vi "DefendGoalTactic.vi"(7 "First call?":bool=TRUE, 8 "error in (no error)":errorcluster, 9 "Robot":refnum<class "Robot.lvclass">, 10 "Game":refnum<class "Game.lvclass">, 11 "DefendGoalTactic in":refnum<class "DefendGoalTactic.lvclass">) -> (0 "error out":errorcluster, 2 "Robot out":refnum<class "Robot.lvclass">, 3 "DefendGoalTactic out":refnum<class "DefendGoalTactic.lvclass">)   [LabVIEW 2024, in "DefendGoalTactic.lvclass"]
uses:
  DefendGoalTactic.lvclass
  Robot_class/Robot.lvclass
  C:/Users/moise/Documents/GitHub/SSL_AI/Object_class/Object.lvclass
  Game_class/Game.lvclass
  C:/Users/moise/Documents/GitHub/SSL_AI/Tactic_class/Tactic.lvclass
  Robot_class/tactics.ctl
  DefendGoalTacticStates.ctl
  Tactic_class/Tactic.lvclass/Tactic.ctl
  Robot_class/robotKickToStates.ctl
  Robot_class/Robot.lvclass/Robot.ctl
  Game_class/Game.lvclass/Game.ctl
  Parameters_class/Parameters.lvclass/Parameters.ctl
  Team_class/Team.lvclass/Team.ctl
  Field_class/Field.lvclass/Field.ctl
  Object_class/Object.lvclass/Object.ctl
  Skillbook_class/Skillbook.lvclass/Skillbook.ctl
  DefendGoalTactic.lvclass/DefendGoalTactic.ctl
  Robot_class/Write robotKickState.vi
  Object_class/Read position(x,y).vi
  Game_class/Read OffensiveTeam.vi
  Game_class/Read EnemyRef.vi
  Game_class/Read Parameters.lvclass.vi
  Game_class/Read Utilities.lvclass.vi
  Game_class/Read FieldRef.vi
  Game_class/Read BallRef.vi
  Field_class/Read ourGoalPosition.vi
  Parameters_class/Read AttakingOurselves.vi
  Team_class/Read RobotRef.vi
  Robot_class/Write dest_orientation.vi
  Robot_class/Write dest_x.vi
  Robot_class/Write dest_y.vi
  Object_class/Read x.vi
  Object_class/Read y.vi
  Game_class/Read NewParameters.vi
  Skillbook_class/Read KickToSkill.vi
  Robot_class/Write kick_x.vi
  Robot_class/Write kick_z.vi
  Tactic_class/Read Skillbook.vi
  Write States.vi
  Robot_class/Write tactic.vi
  Robot_class/Write keepDest.vi
  Enemy_class/Enemy.lvclass
  C:/Users/moise/Documents/GitHub/SSL_AI/Team_class/Team.lvclass
  Ally_class/Ally.lvclass
  Ball_class/Ball.lvclass
  Skillbook_class/Skillbook.lvclass
  DefBallTrajSkill_class/DefBallTrajSkill.lvclass
  Parameters_class/Parameters.lvclass
  Utilities_class/Utilities.lvclass
  Field_class/Field.lvclass
  KickToSkill_class/KickToSkill.lvclass
  ShootTactic_class/ShootTactic.lvclass
  <vilib>/Analysis/NI_AALPro.lvlib
  <vilib>/Analysis/coordinate.llb/2D Cartesian Coordinate Rotation (Scalar).vi
  Team_class/Team.lvclass
  DefBallEnemySkill_class/DefBallEnemySkill.lvclass
  DefBallOrientSkill_class/DefBallOrientSkill.lvclass
panel:
  out "Dist":dbl
  out "x .or. y?":bool
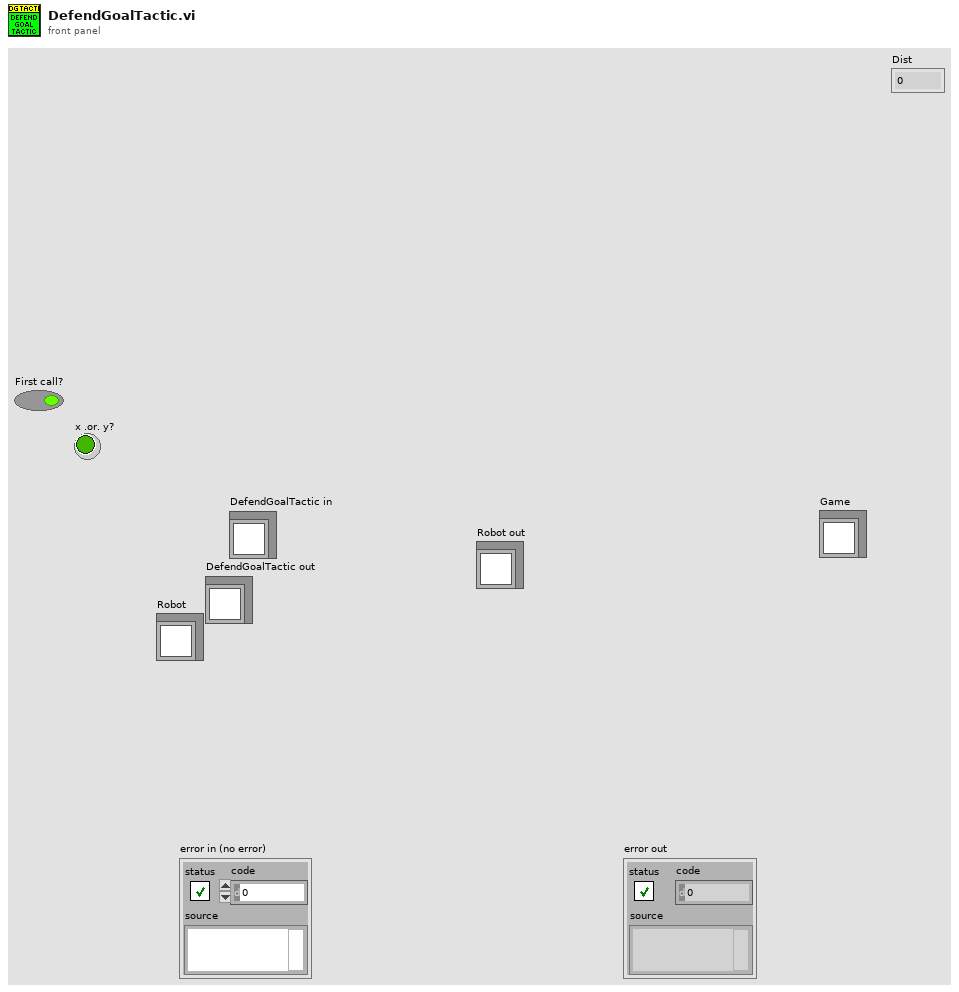
[diagram p1: front panel]
types:
  T1 = typedef "DefendGoalTactic.lvclass/DefendGoalTacticStates.ctl" = enum16{"BlockShot", "BlockPossibleShot", "CoverOneTouchShot", "Kick", "GuardGoal", "Exit"}
  T2 = typedef "tactics.ctl" = enum16{"GoToBallPlacementPosition", "PlaceBall", "GoToBallPlacement", "5Robots", "BallPlacementEnemy", "ReceivePassInFuturePoint", "Roller", "PrepareRollToPassRollerGoTo", "PrepareRollToPassReceiverGoTo", "WaitRoll", "PositionToRoll", "PenaltyAttacker", "PassObserver", "PenaltyDefense", "TableReceiverTactic", "Test", "DefendGoal", "Marker", "FollowAttacker", "DefendArea", "Shoot", "AttackerAimGoal", "AttackerBallOutOfField", "AttackerBlock", "AttackerStop", "Duelist", "Halt", "ZigZag", "GoTo", "Timeout", "KickToBestRobot", "KickToPassReceiver", "PositionToReceivePass", "WaitPass", "GoToTarget"}
  T3 = typedef "robotKickToStates.ctl" = enum16{"shootFromDirect", "avoidCollideBall", "goToBackBall", "none", "walk", "turn", "turnAntiClockWise", "turnClockwise", "oldKickToShoot", "oldKickToGoToBackBall", "shoot"}
  T4 = typedef "NewParameters.ctl" = cluster{"PenaltyDistance":dbl, "DistanceAttackerToBackBall":dbl, "Division":enum16{"Div B", "Div A"}, "DistanceToAvoidyEnemyRobot":dbl, "BallPlacementDistance":dbl, "DisatanceBehindBallToStealBall":dbl, "MaxDistanceToPositionKickoff":dbl, "BlockEnemyTarget":bool, "MaxStopVAng":dbl, "DistanceMarkerToEnemy":dbl, "IgnoreDribblerContact":bool, "DistanceToBeginEnemyPosession":dbl, "GoToBallWhenEnemyNotMoving":bool, "EnemyDistanceToReduceVelocity":dbl, "TurnOnEnemyDistanceToReduceVelocity":bool, "EnemyDistanceToShootOutBall":dbl, "DefenseKickBall":bool, "MoreKickToGoal? (0-0.3)":dbl, "ChipKickInEnemyField":bool, "ShootOutRobotId":dbl, "FieldLenghtDenominatorInShootOut":dbl, "AdjustPositionInBallPlacement":bool, "PowerGodPass":dbl, "VelocityAbortEnemyPos":dbl, "MaxDistToBeginPass":dbl, "MinDistToBeginPass":dbl, "VelocityInDirects":dbl, "BadDribblerIDs":i32[], "NewKickToDistanceAroundBall":dbl, "PowerAvoidColisionMarker":dbl, "DistanceToAvoidColisionMarker":dbl, "AvoidBallKick":dbl, "DistanceTryKick":dbl, "SuicideKickDIstance":dbl, "AdjustFirstKickDistance":dbl, "AvoidAimLessKick":dbl, "DistanceToAvoidyEnemyShootRobot ":dbl, "NumberOfMarkers":dbl, "PotField":bool, "PIDLateral":bool, "MinDistanceFirstKickX":dbl, "MinDistanceFirstKickY":dbl, "FractionOfDistToTouchGround\nAfterChipKick":dbl, "FractionOfKickxWhen\nComposedWithKickz":dbl, "Style":T5, "MoveInTurnState":bool, "DistFromEnemyToConsider\nMoveInTurnState":dbl, "CascadePID":bool, "TurnAroundParameters":cluster{"Radius":dbl, "Multiplier":dbl, "ChordAngle":dbl}, "SafeDriveVel":dbl, "DistanceToGoToBackBall":dbl, "minDistanceToNotFinish\nEnemyPossession":dbl, "OneTouchShot":cluster{"angleFactor":dbl, "maxAngle":dbl, "Attack":bool, "Defense":bool}, "OpenAngleToGoal":cluster{"minAngle":dbl, "maxAngle":dbl, "minEvaluation":dbl}, "ShotInterception":cluster{"shotSpeed":dbl, "minEnemySpeed":dbl, "maxEnemySpeed":dbl, "minEvaluation":dbl}, "AllyTeamArray":T6[], "maxDefendersNumber":i32, "Zone":cluster{"GuardPositionArray":dbl[][], "ZoneMidField":dbl[], "CenterForwardWidth":dbl}, "MinEvaluationToShoot":dbl, "PassInterception":cluster{"maxPassSpeed":dbl, "minPassSpeed":dbl, "minEnemySpeed":dbl, "chipPassDistance":dbl, "chipPassEvaluation":dbl, "minEvaluation":dbl, "maxEnemySpeed":dbl}, "PassDistance":cluster{"maxDistance":dbl, "minDistance":dbl}, "receiverSpeed":dbl, "maxBallSpeed":dbl, "slackTime":dbl, "Turning radius":dbl, "Turning v_ang":dbl, "AlignError":cluster{"Distance":dbl, "Orientation":dbl, "V_norm(m/s)":dbl, "V_ang (rad/s)":dbl}, "RobotRadius":dbl, "KickerDistance":dbl, "keeper angle  to cover goalpost":dbl, "a_slide":dbl, "a_roll":dbl, "k_switch":dbl}
  T5 = typedef "Style.ctl" = enum16{"Insanity", "Offensive", "Defensive"}
  T6 = typedef "AllyTeam.ctl" = enum16{"Keeper", "Defender", "Attacker"}
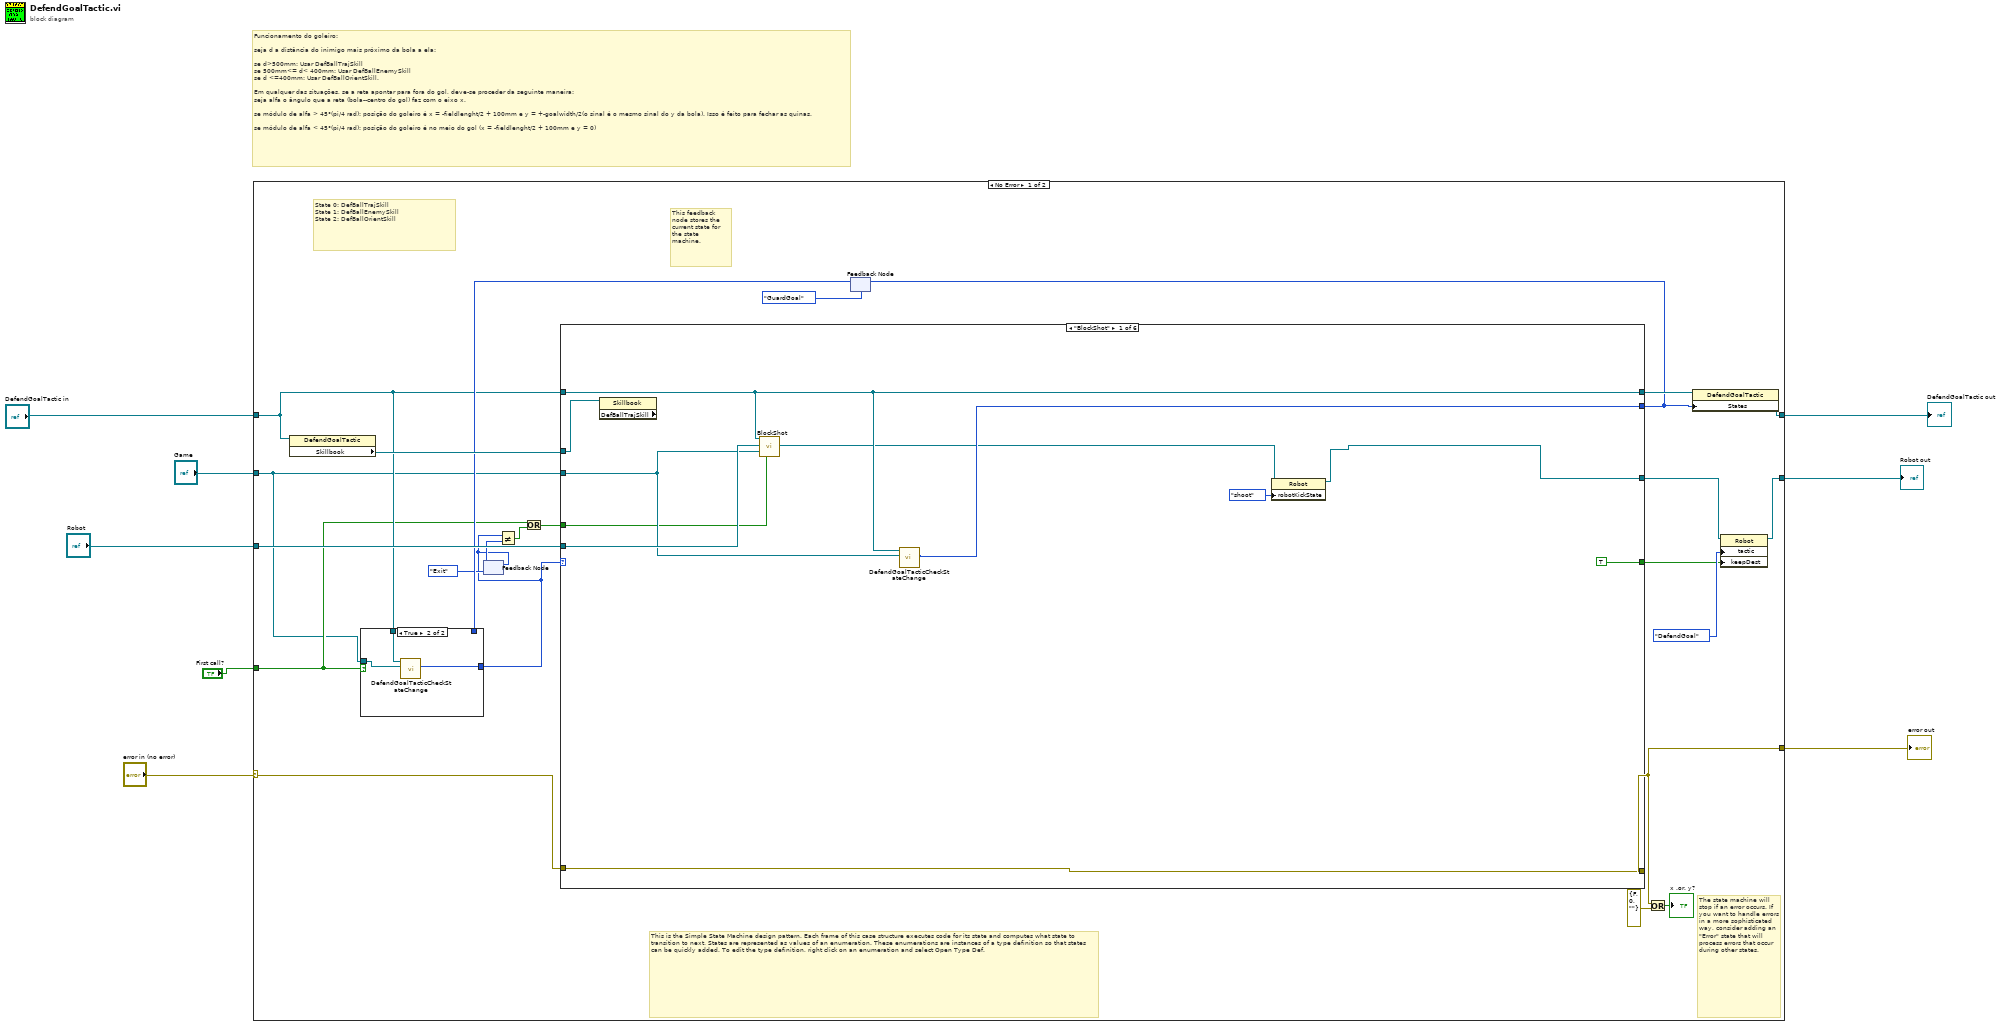
[diagram p0: block diagram]
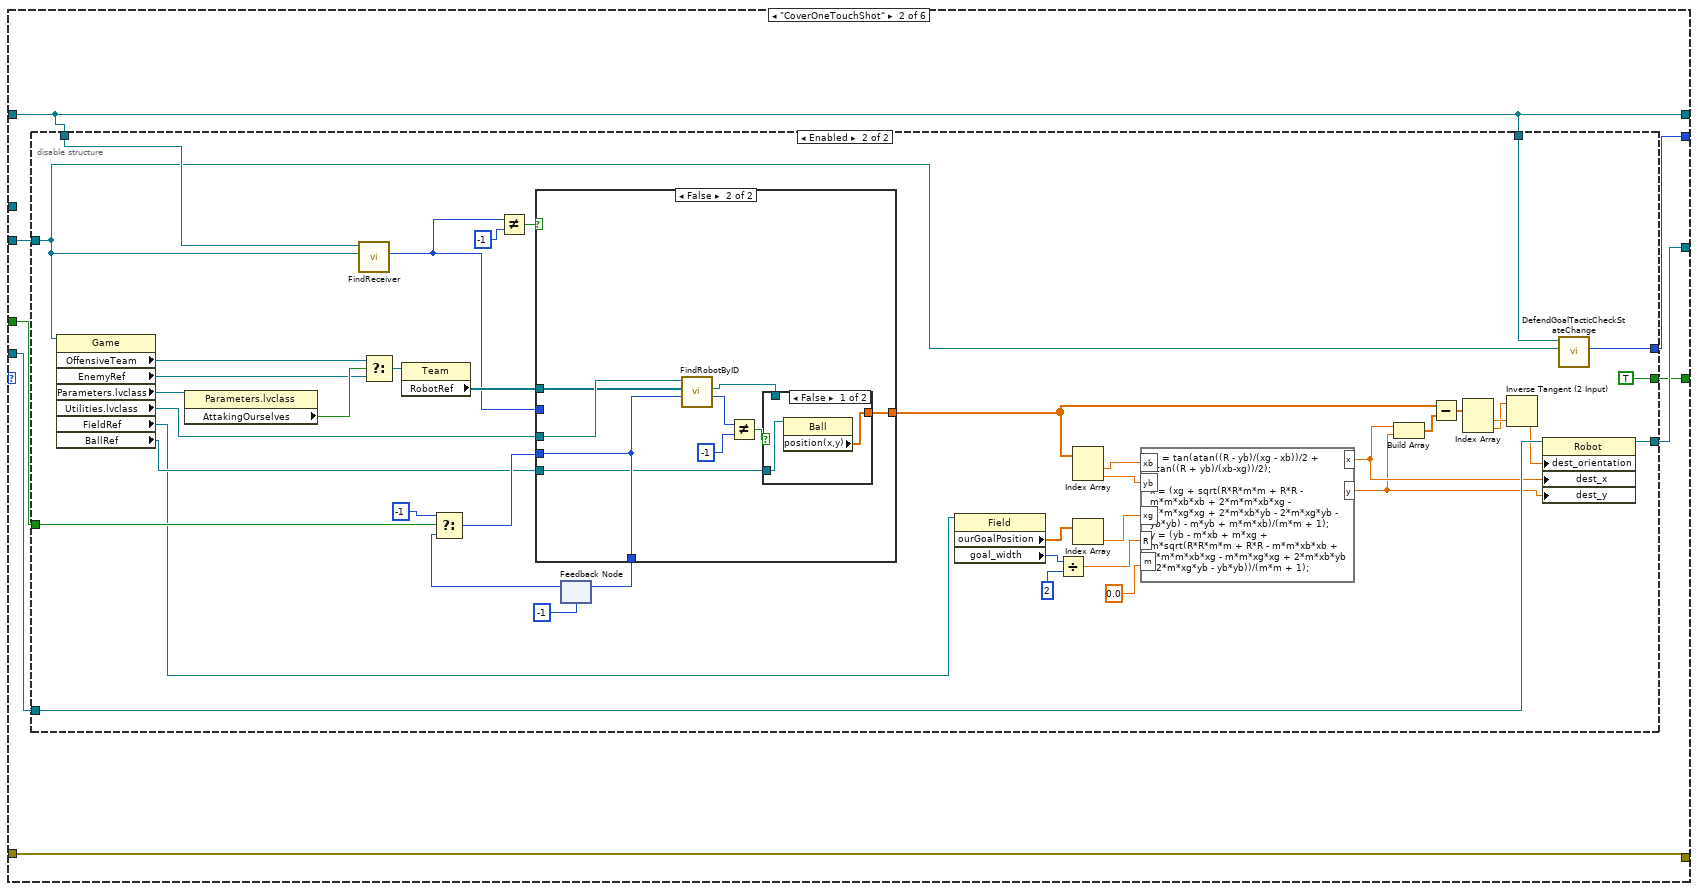
[diagram p3: hidden frame]
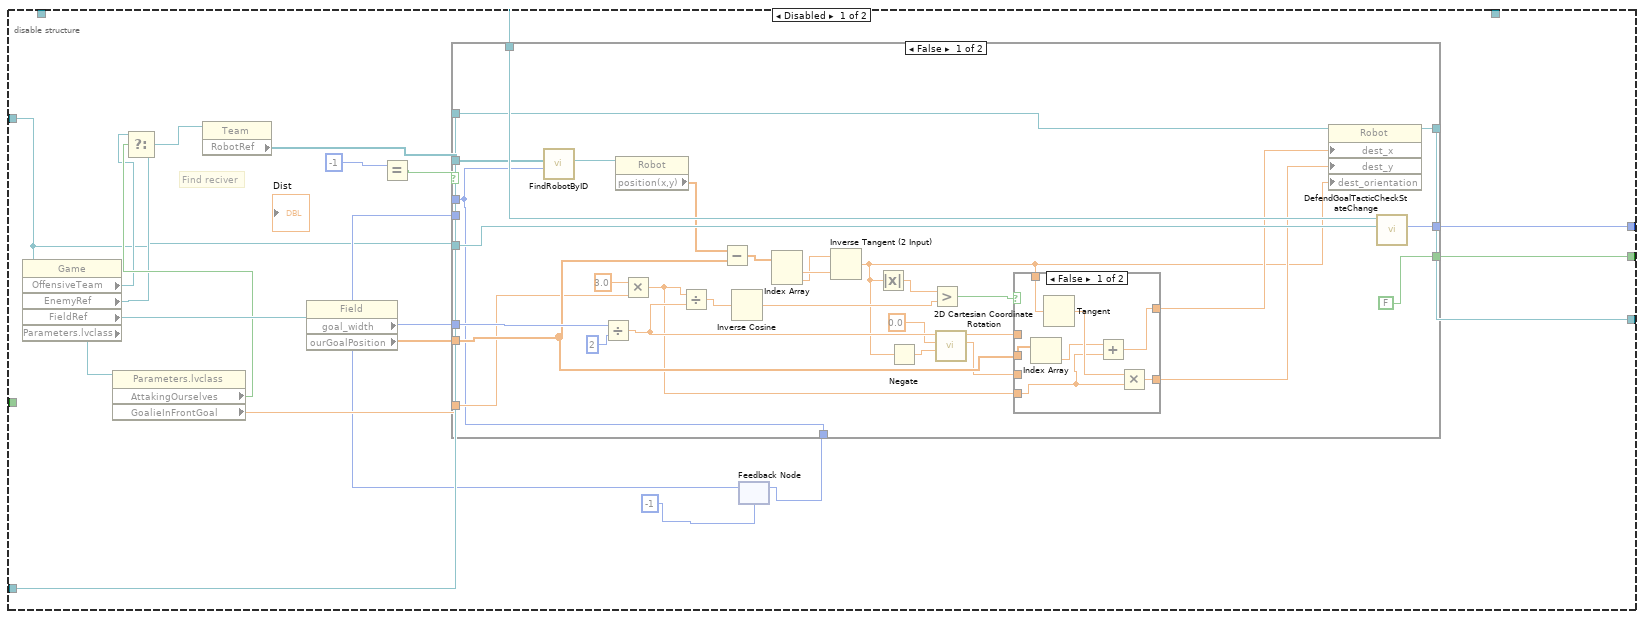
[diagram p4: hidden frame]
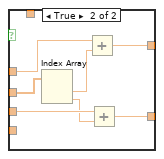
[diagram p5: hidden frame]
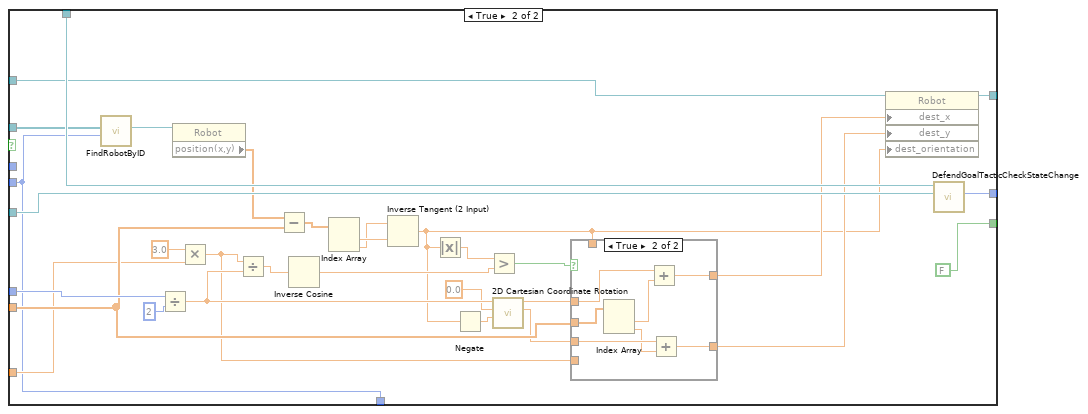
[diagram p6: hidden frame]
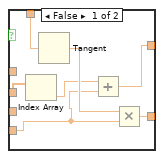
[diagram p7: hidden frame]
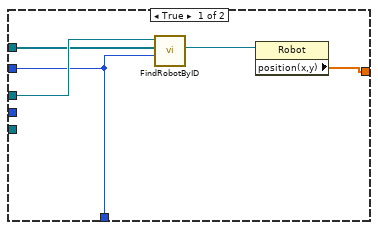
[diagram p8: hidden frame]
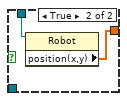
[diagram p9: hidden frame]
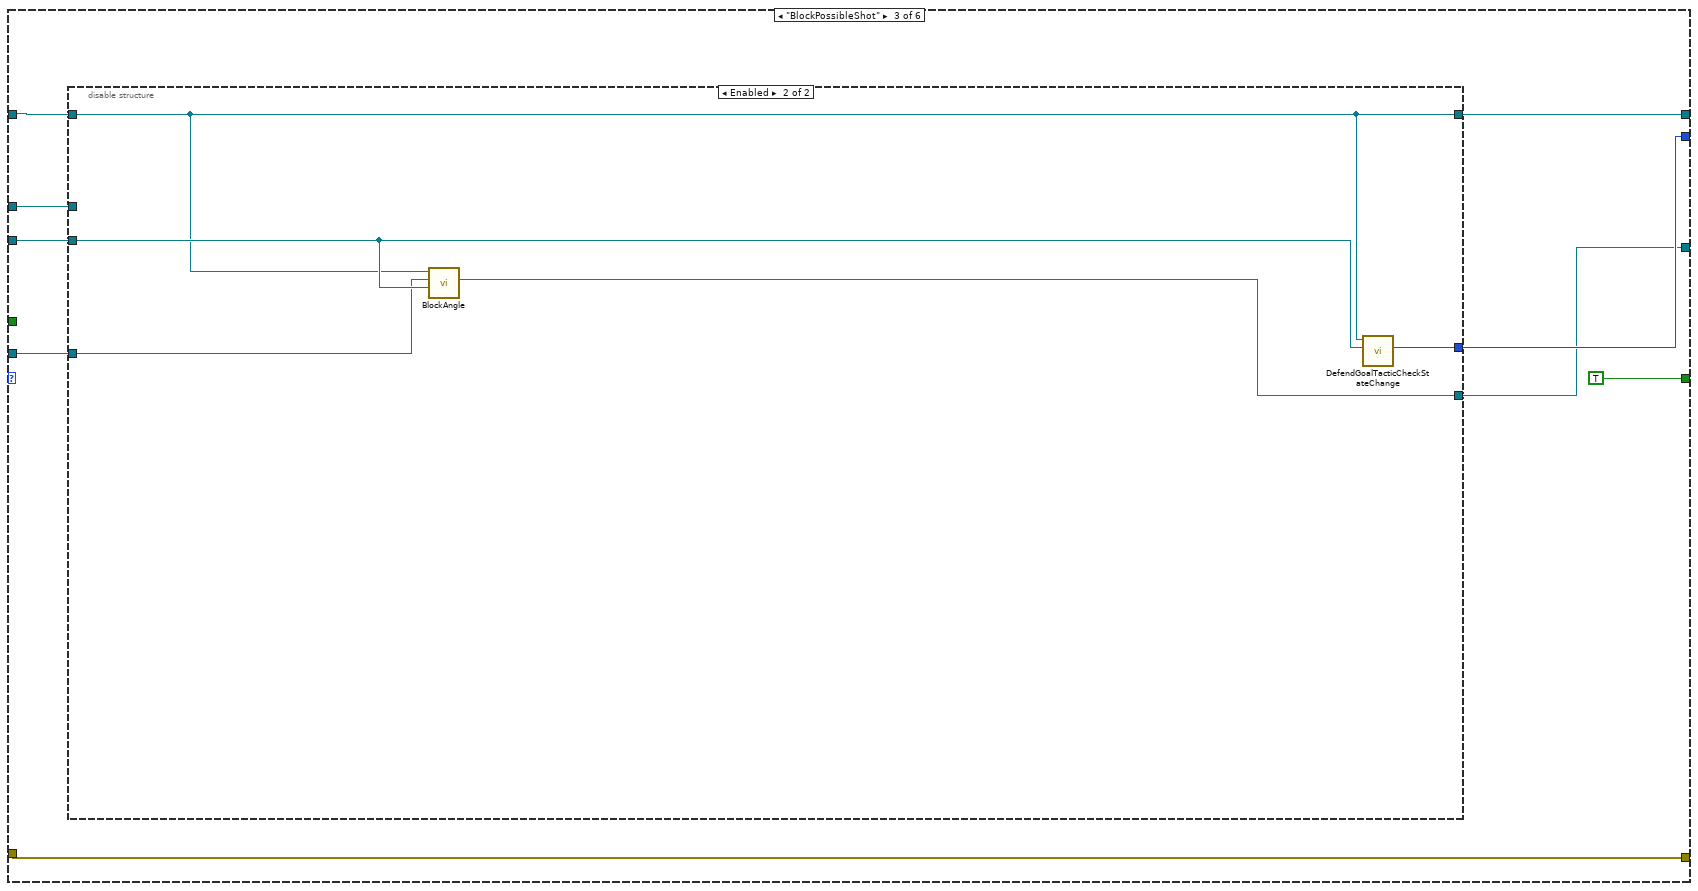
[diagram p10: hidden frame]
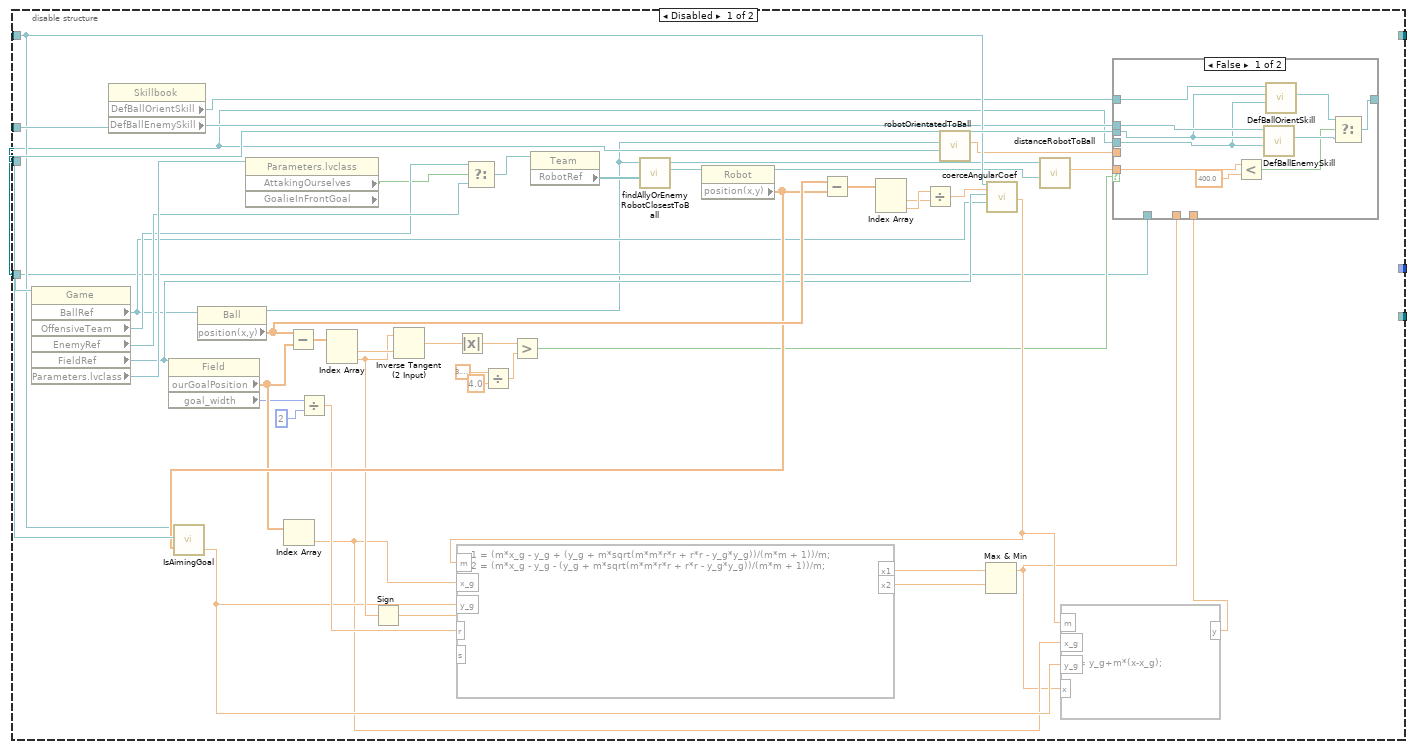
[diagram p11: hidden frame]
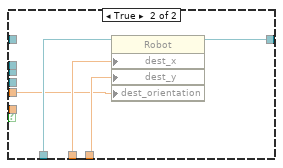
[diagram p12: hidden frame]
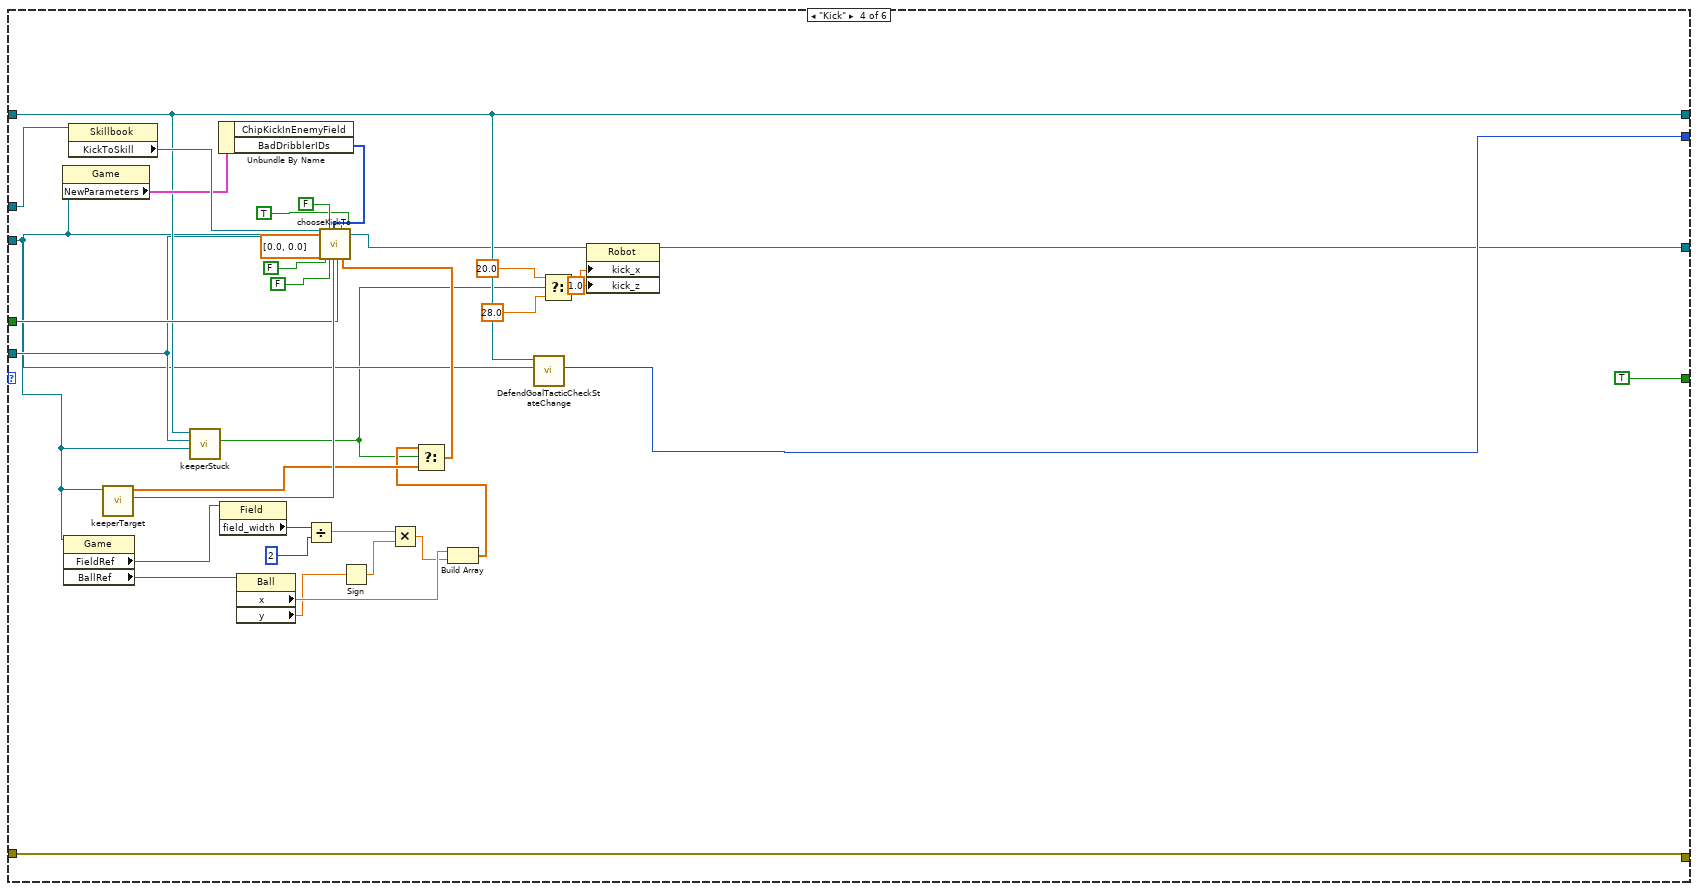
[diagram p13: hidden frame]
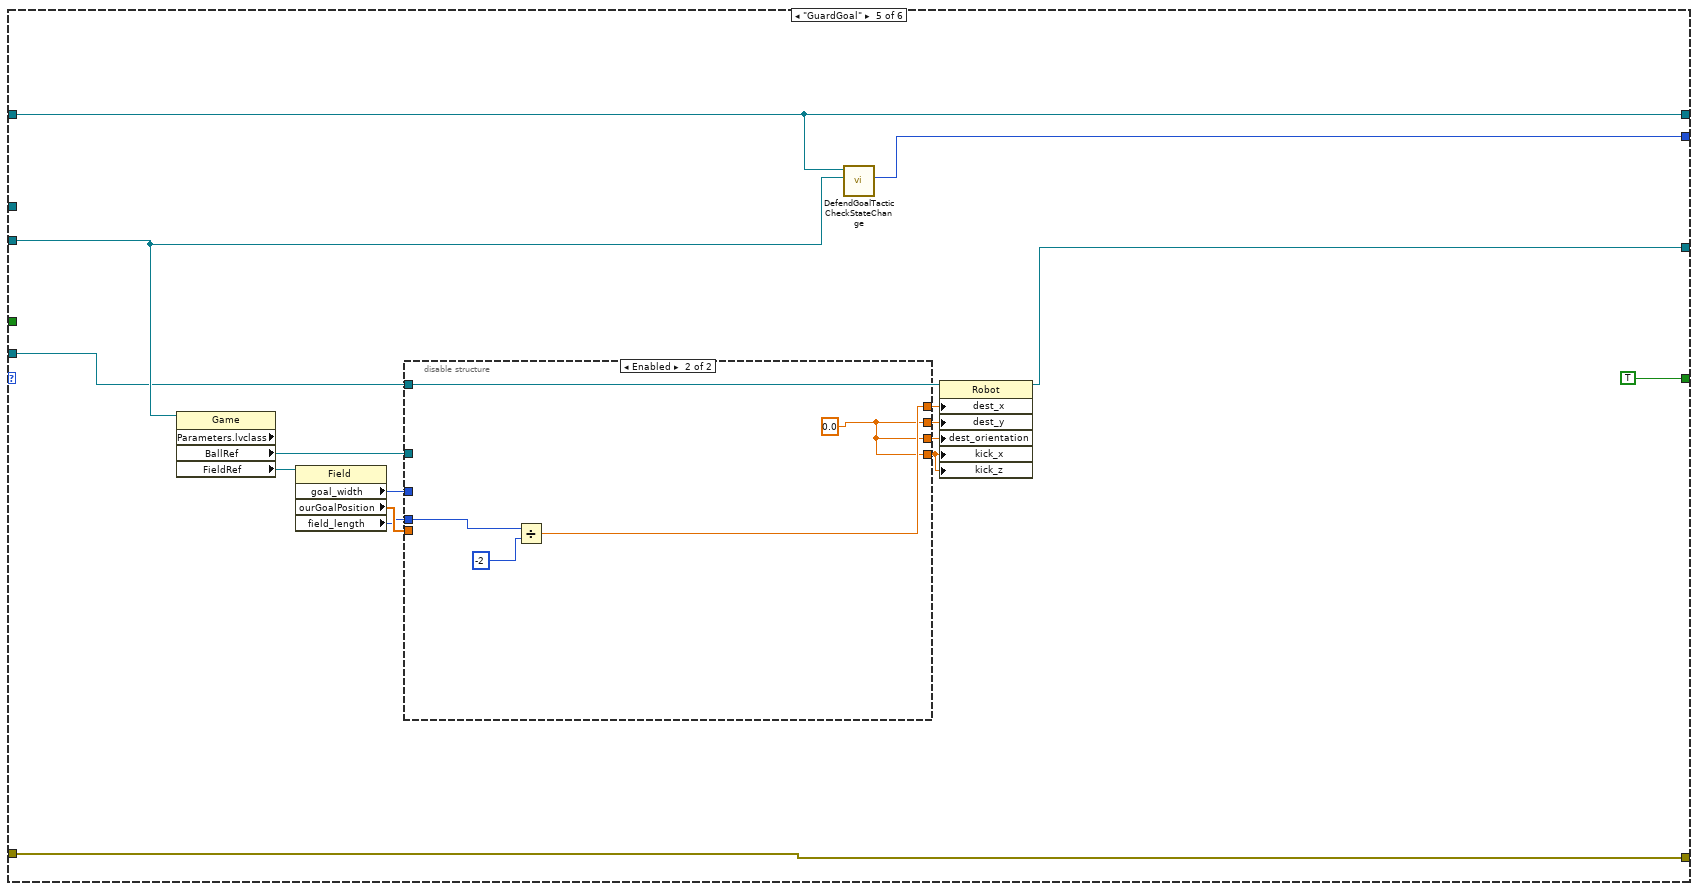
[diagram p14: hidden frame]
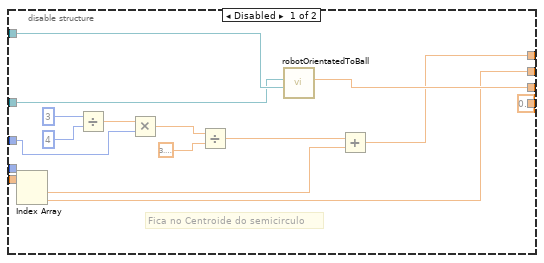
[diagram p15: hidden frame]
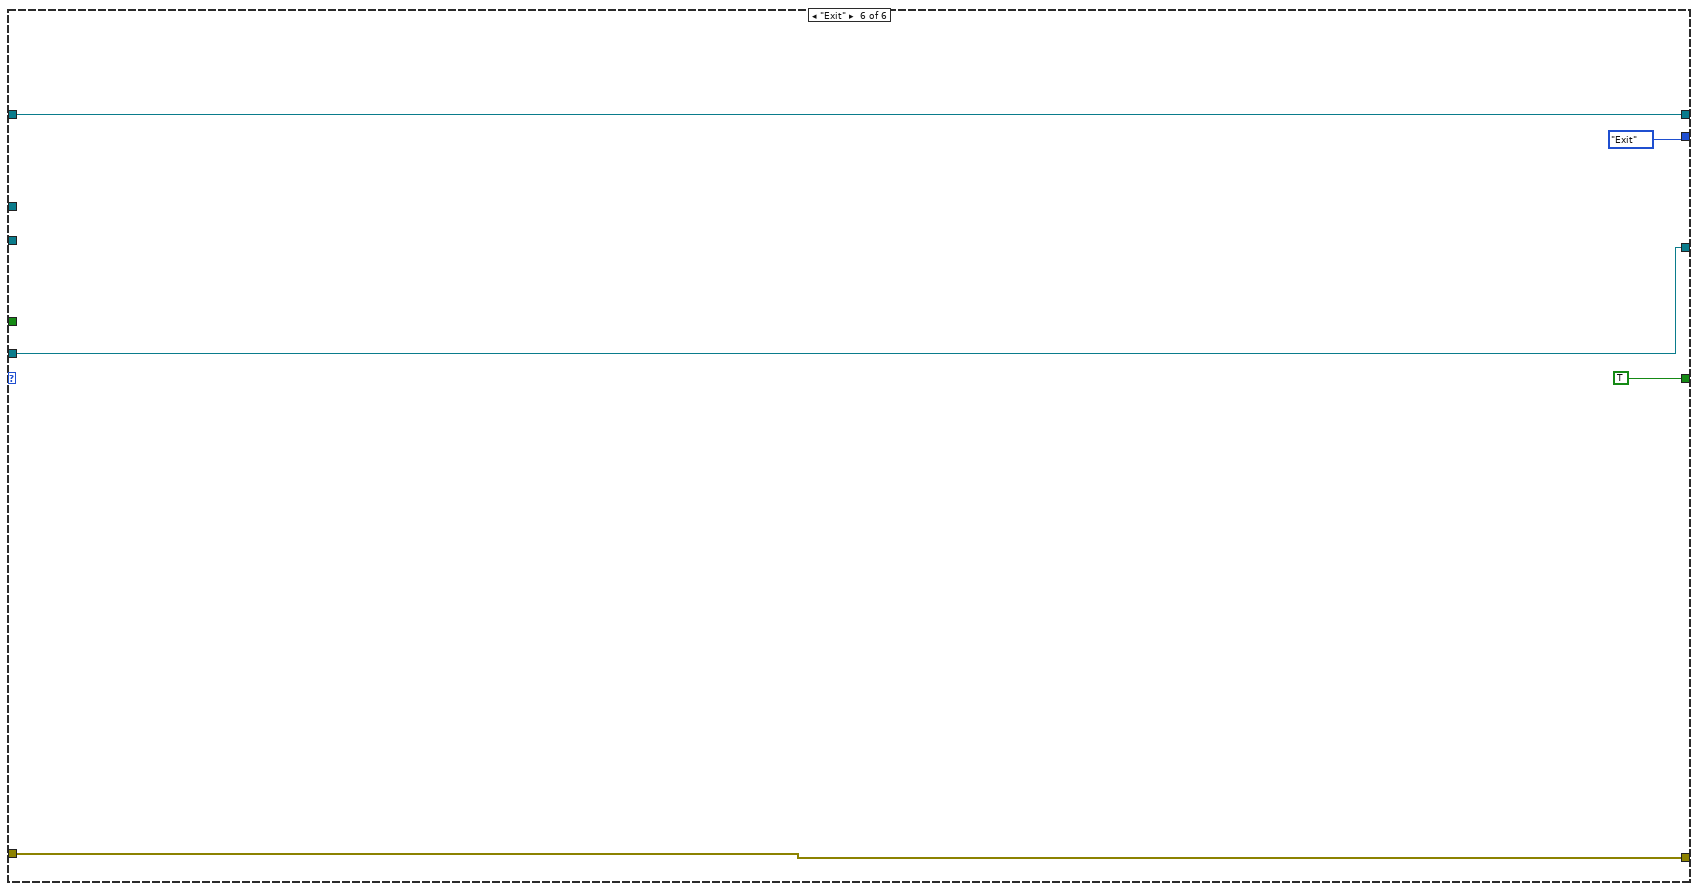
[diagram p16: hidden frame]
diagram:
  # "Funcionamento do goleiro:\n\nseja d a distância do inimigo mais próximo da bola a ela:\n\nse d>500mm: Usar DefBallTrajSkill\nse 500mm<= d< 400mm: Usar DefBallEnemySkill\nse d <=400mm: Usar DefBallOrientSkill.\n\nEm qualquer das situações, se a reta apontar para fora do gol, deve-se proceder da seguinte maneira:\nseja alfa o ângulo que a reta (bola--centro do gol) faz com o eixo x.\n\nse módulo de alfa > 45°(pi/4 rad): posição do goleiro é x = -fieldlenght/2 + 100mm e y = +-goalwidth/2(o sinal é o mesmo sinal do y da bola). Isso é feito para fechar as quinas.\n\nse módulo de alfa < 45°(pi/4 rad): posição do goleiro é no meio do gol (x = -fieldlenght/2 + 100mm e y = 0)"
  n1 = case shown="No Error" "error in (no error)" {
    selector: "error in (no error)" -> [w30 w378]
    tunnel: [w29 w378] -> w7
    tunnel: [w25 w377] -> w2
    tunnel: "DefendGoalTactic in" -> [w22 w377]
    tunnel: "Robot" -> [w28 w376]
    tunnel: [w19 w376] -> w5
    tunnel: "Game" -> [w10 _]
    tunnel: "First call?" -> [w16 _]
    frame No Error {
      # "State 0: DefBallTrajSkill\nState 1: DefBallEnemySkill\nState 2: DefBallOrientSkill"
      # "The state machine will stop if an error occurs. If you want to handle errors in a more sophisticated way, consider adding an \"Error\" state that will process errors that occur during other states."
      # "This feedback node stores the current state for the state machine."
      # "This is the Simple State Machine design pattern. Each frame of this case structure executes code for its state and computes what state to transition to next. States are represented as values of an enumeration. These enumerations are instances of a type definition so that states can be quickly added. To edit the type definition, right click on an enumeration and select Open Type Def."
      n2 = property class="DefendGoalTactic"(reference=w22) -> ("Skillbook"=w27:refnum<class "Skillbook.lvclass">)  [unwired: 1 in, 2 out]
      n3 = feedback #1(DefendGoalTacticStates."Exit" ("States")) -> (w14:T1)
      n4 = feedback #2(DefendGoalTacticStates."GuardGoal" ("States")) -> (w24:T1)
      n5 = case shown="True" w16 {
        tunnel: [w32 w35] -> w9
        tunnel: w24 -> [w32 _]
        tunnel: w10 -> [_ w34]
        tunnel: w22 -> [_ w33]
        frame False {
        }
        frame True {
          n6 = call "DefendGoalTacticCheckStateChange.vi"("Game"=w34, "DefendGoalTactic in"=w33) -> ("States"=w35:T1)  [unwired: 7 in, 2 out]
        }
      }
      n7 = feedback-in #1(w9) -> ()
      n8 = Not Equal?(x=w9, y=w14) -> (x != y?=w15:bool)
      n9 = Or(x=w16, y=w15) -> (x .or. y?=w17:bool)
      n10 = case shown="\"BlockShot\"" w9 {
        tunnel: w30 -> [w46 w54 w233 w335 w351 w375]
        tunnel: [w46 w54 w233 w335 w351 w375] -> w29
        tunnel: w27 -> [w45 _ w232 w333 _ _]
        tunnel: w28 -> [w41 w51 w230 w320 w346 w371]
        tunnel: [w37 w52 w227 w306 w344 w371] -> w20
        tunnel: [w42 w48 w225 w324 w349 w372] -> w26
        tunnel: w22 -> [w42 w48 w229 w324 w349 w372]
        tunnel: w10 -> [w40 w53 w231 w319 w348 _]
        tunnel: [w44 w49 w228 w308 w350 DefendGoalTacticStates."Exit" ("States")] -> w18
        tunnel: w17 -> [w39 w47 _ w329 _ _]
        tunnel: [TRUE ("keepDest") w50 TRUE TRUE ("keepDest") TRUE ("keepDest") TRUE ("keepDest")] -> w11
        frame "BlockShot" {
          n11 = property class="Skillbook" props=["DefBallTrajSkill"](reference=w45) -> ()  [unwired: 1 in, 3 out]
          n12 = call "BlockShot.vi"("object in"=w42, "Robot"=w41, "Game"=w40, "first call?"=w39) -> ("Robot out"=w38:refnum<class "Robot.lvclass">)  [unwired: 13 in, 2 out]
          n13 = call "DefendGoalTacticCheckStateChange.vi"("Game"=w40, "DefendGoalTactic in"=w42) -> ("States"=w44:T1)  [unwired: 7 in, 2 out]
          n14 = property class="Robot"(reference=w38, "robotKickState"=robotKickToStates."shoot") -> (reference out=w37:refnum<class "Robot.lvclass">)  [unwired: 1 in, 1 out]
        }
        frame "CoverOneTouchShot" {
          n15 = disable-structure shown="Enabled" {
            disable-tunnel: w48 -> [w75 w202]
            disable-tunnel: w53 -> [w55 w191]
            disable-tunnel: [w73 w186] -> w52
            disable-tunnel: w51 -> [w72 w173]
            disable-tunnel: [w67 w195] -> w49
            disable-tunnel: [w63 TRUE ("keepDest")] -> w50
            disable-tunnel: w48 -> [_ w194]
            disable-tunnel: w47 -> [_ w190]
            frame Disabled {
              # "Find reciver"
              n16 = property class="Game"(reference=w55) -> ("OffensiveTeam"=w56:refnum<class "Ally.lvclass">, "EnemyRef"=w57:refnum<class "Enemy.lvclass">, "FieldRef"=w71:refnum<class "Field.lvclass">, "Parameters.lvclass"=w65:refnum<class "Parameters.lvclass">)  [unwired: 1 in, 2 out]
              n17 = property class="Parameters.lvclass"(reference=w65) -> ("AttakingOurselves"=w59:bool, "GoalieInFrontGoal"=w64:dbl)  [unwired: 1 in, 2 out]
              n18 = Select(t=w56, s=w59, f=w57) -> (s? t:f=w58:refnum<class "Team.lvclass">)
              n19 = property class="Team"(reference=w58) -> ("RobotRef"=w74:refnum<class "Robot.lvclass">[])  [unwired: 1 in, 2 out]
              n20 = property class="Field"(reference=w71) -> ("goal_width"=w66:i32, "ourGoalPosition"=w70:dbl[])  [unwired: 1 in, 2 out]
              n21 = Equal?(x=-1) -> (x = y?=w68:bool)  [unwired: 1 in]
              n22 = feedback #3(-1 ("x")) -> (w61:i32)
              n23 = case shown="False" w68 {
                tunnel: w75 -> [w106 w151]
                tunnel: w55 -> [w105 w150]
                tunnel: w74 -> [w104 w149]
                tunnel: [w103 w148] -> w73
                tunnel: w72 -> [w102 w147]
                tunnel: w70 -> [w86 w131]
                tunnel: [w100 w145] -> w67
                tunnel: w66 -> [w95 w140]
                tunnel: w64 -> [w84 w129]
                tunnel: _ -> [w78 _]
                tunnel: [FALSE ("keepDest") FALSE ("keepDest")] -> w63
                tunnel: w61 -> [_ w123]
                tunnel: [w78 w123] -> w60
                frame False {
                  n24 = call "FindRobotByID.vi"("id"=w78, "RobotRef"=w104) -> ("Robot"=w101:refnum<class "Robot.lvclass">)  [unwired: 6 in, 3 out]
                  n25 = Divide(x=w95, y=2) -> (x/y=w88:dbl)
                  n26 = property class="Robot"(reference=w101) -> ("position(x,y)"=w99:dbl[])  [unwired: 1 in, 2 out]
                  n27 = Multiply(x=3.0, y=w84) -> (x*y=w80:dbl)
                  n28 = Divide(x=w80, y=w88) -> (x/y=w92:dbl)
                  n29 = Subtract(x=w99, y=w86) -> (x-y=w98:dbl[])
                  n30 = Inverse Cosine(1:w92) -> (0:w91:dbl)
                  n31 = Index Array(array=w98) -> (element #1=w97:dbl, element #2=w96:dbl)  [unwired: 2 in]
                  n32 = Inverse Tangent (2 Input)(1:w97, 2:w96) -> (0:w77:dbl)
                  n33 = Absolute Value(x=w77) -> (abs(x)=w90:dbl)
                  n34 = Negate(x=w77) -> (-x=w76:dbl)
                  n35 = Greater?(x=w90, y=w91) -> (0:w89:bool)
                  n36 = call-poly <vilib>:"2D Cartesian Coordinate Rotation.vi"("theta"=w76, "y"=0.0 ("element"), "x"=w88) -> ("y out"=w83:dbl, "x out"=w85:dbl)  [unwired: 6 in, 1 out]
                  n37 = case shown="False" w89 {
                    tunnel: w86 -> [w110 w118]
                    tunnel: w85 -> [_ w120]
                    tunnel: w83 -> [_ w119]
                    tunnel: [w107 w115] -> w82
                    tunnel: [w111 w114] -> w81
                    tunnel: w80 -> [w108 _]
                    tunnel: w77 -> [w113 _]
                    frame False {
                      n38 = Index Array(array=w110) -> (element=w109:dbl)  [unwired: 1 in]
                      n39 = Tangent(1:w113) -> (0:w112:dbl)
                      n40 = Add(x=w109, y=w108) -> (x+y=w107:dbl)
                      n41 = Multiply(x=w112, y=w108) -> (x*y=w111:dbl)
                    }
                    frame True {
                      n42 = Index Array(array=w118) -> (element #1=w117:dbl, element #2=w116:dbl)  [unwired: 2 in]
                      n43 = Add(x=w120, y=w117) -> (x+y=w115:dbl)
                      n44 = Add(x=w119, y=w116) -> (x+y=w114:dbl)
                    }
                  }
                  n45 = property class="Robot"(reference=w102, "dest_x"=w82, "dest_y"=w81, "dest_orientation"=w77) -> (reference out=w103:refnum<class "Robot.lvclass">)  [unwired: 1 in, 1 out]
                  n46 = call "DefendGoalTacticCheckStateChange.vi"("Game"=w105, "DefendGoalTactic in"=w106) -> ("States"=w100:T1)  [unwired: 7 in, 2 out]
                }
                frame True {
                  n47 = call "FindRobotByID.vi"("id"=w123, "RobotRef"=w149) -> ("Robot"=w146:refnum<class "Robot.lvclass">)  [unwired: 6 in, 3 out]
                  n48 = Divide(x=w140, y=2) -> (x/y=w133:dbl)
                  n49 = property class="Robot"(reference=w146) -> ("position(x,y)"=w144:dbl[])  [unwired: 1 in, 2 out]
                  n50 = Multiply(x=3.0, y=w129) -> (x*y=w125:dbl)
                  n51 = Divide(x=w125, y=w133) -> (x/y=w137:dbl)
                  n52 = Subtract(x=w144, y=w131) -> (x-y=w143:dbl[])
                  n53 = Inverse Cosine(1:w137) -> (0:w136:dbl)
                  n54 = Index Array(array=w143) -> (element #1=w142:dbl, element #2=w141:dbl)  [unwired: 2 in]
                  n55 = Inverse Tangent (2 Input)(1:w142, 2:w141) -> (0:w122:dbl)
                  n56 = Absolute Value(x=w122) -> (abs(x)=w135:dbl)
                  n57 = Negate(x=w122) -> (-x=w121:dbl)
                  n58 = Greater?(x=w135, y=w136) -> (0:w134:bool)
                  n59 = call-poly <vilib>:"2D Cartesian Coordinate Rotation.vi"("theta"=w121, "y"=0.0 ("element"), "x"=w133) -> ("y out"=w128:dbl, "x out"=w130:dbl)  [unwired: 6 in, 1 out]
                  n60 = case shown="True" w134 {
                    tunnel: w131 -> [w155 w163]
                    tunnel: w130 -> [_ w165]
                    tunnel: w128 -> [_ w164]
                    tunnel: [w152 w160] -> w127
                    tunnel: [w156 w159] -> w126
                    tunnel: w125 -> [w153 _]
                    tunnel: w122 -> [w158 _]
                    frame False {
                      n61 = Index Array(array=w155) -> (element=w154:dbl)  [unwired: 1 in]
                      n62 = Tangent(1:w158) -> (0:w157:dbl)
                      n63 = Add(x=w154, y=w153) -> (x+y=w152:dbl)
                      n64 = Multiply(x=w157, y=w153) -> (x*y=w156:dbl)
                    }
                    frame True {
                      n65 = Index Array(array=w163) -> (element #1=w162:dbl, element #2=w161:dbl)  [unwired: 2 in]
                      n66 = Add(x=w165, y=w162) -> (x+y=w160:dbl)
                      n67 = Add(x=w164, y=w161) -> (x+y=w159:dbl)
                    }
                  }
                  n68 = property class="Robot"(reference=w147, "dest_x"=w127, "dest_y"=w126, "dest_orientation"=w122) -> (reference out=w148:refnum<class "Robot.lvclass">)  [unwired: 1 in, 1 out]
                  n69 = call "DefendGoalTacticCheckStateChange.vi"("Game"=w150, "DefendGoalTactic in"=w151) -> ("States"=w145:T1)  [unwired: 7 in, 2 out]
                }
              }
              n70 = feedback-in #3(w60) -> ()
            }
            frame Enabled {
              n71 = property class="Game"(reference=w191) -> ("OffensiveTeam"=w204:refnum<class "Ally.lvclass">, "EnemyRef"=w203:refnum<class "Enemy.lvclass">, "Parameters.lvclass"=w206:refnum<class "Parameters.lvclass">, "Utilities.lvclass"=w201:refnum<class "Utilities.lvclass">, "FieldRef"=w171:refnum<class "Field.lvclass">, "BallRef"=w172:refnum<class "Ball.lvclass">)  [unwired: 1 in, 2 out]
              n72 = property class="Parameters.lvclass"(reference=w206) -> ("AttakingOurselves"=w205:bool)  [unwired: 1 in, 2 out]
              n73 = call "FindReceiver.vi"("Game"=w191, "object in"=w202) -> ("Receiver Id"=w197:i32)  [unwired: 6 in, 3 out]
              n74 = Select(t=w204, s=w205, f=w203) -> (s? t:f=w200:refnum<class "Team.lvclass">)
              n75 = property class="Team"(reference=w200) -> ("RobotRef"=w199:refnum<class "Robot.lvclass">[])  [unwired: 1 in, 2 out]
              n76 = Not Equal?(x=w197, y=-1) -> (x != y?=w198:bool)
              n77 = feedback #4(-1 ("Receiver Id")) -> (w188:i32)
              n78 = Select(t=-1 ("Receiver Id"), s=w190, f=w188) -> (s? t:f=w187:i32)
              n79 = case shown="False" w198 {
                tunnel: w197 -> [w209 _]
                tunnel: w201 -> [w211 w220]
                tunnel: w199 -> [w210 w219]
                tunnel: [w209 w218] -> w193
                tunnel: w187 -> [_ w218]
                tunnel: [w207 w213] -> w167
                tunnel: w172 -> [_ w212]
                frame True {
                  n80 = call "FindRobotByID.vi"("id"=w209, "RobotRef"=w210, "Utilities in"=w211) -> ("Robot"=w208:refnum<class "Robot.lvclass">)  [unwired: 5 in, 3 out]
                  n81 = property class="Robot"(reference=w208) -> ("position(x,y)"=w207:dbl[])  [unwired: 1 in, 2 out]
                }
                frame False {
                  n82 = call "FindRobotByID.vi"("id"=w218, "RobotRef"=w219, "Utilities in"=w220) -> ("index"=w216:i32, "Robot"=w214:refnum<class "Robot.lvclass">)  [unwired: 5 in, 2 out]
                  n83 = Not Equal?(x=w216, y=-1) -> (x != y?=w217:bool)
                  n84 = case shown="False" w217 {
                    tunnel: w214 -> [_ w224]
                    tunnel: [w221 w223] -> w213
                    tunnel: w212 -> [w222 _]
                    frame False {
                      n85 = property class="Ball"(reference=w222) -> ("position(x,y)"=w221:dbl[])  [unwired: 1 in, 2 out]
                    }
                    frame True {
                      n86 = property class="Robot"(reference=w224) -> ("position(x,y)"=w223:dbl[])  [unwired: 1 in, 2 out]
                    }
                  }
                }
              }
              n87 = feedback-in #4(w193) -> ()
              n88 = property class="Field"(reference=w171) -> ("ourGoalPosition"=w183:dbl[], "goal_width"=w181:i32)  [unwired: 1 in, 2 out]
              n89 = Divide(x=w181, y=2) -> (x/y=w179:dbl)
              n90 = Index Array(array=w167) -> (element #1=w185:dbl, element #2=w184:dbl)  [unwired: 2 in]
              n91 = Index Array(array=w183) -> (element=w182:dbl)  [unwired: 1 in]
              n92 = formula code="m = tan(atan((R - yb)/(xg - xb))/2 + atan((R + yb)/(xb-xg))/2);\n\nx = (xg + sqrt(R*R*m*m + R*R - m*m*xb*xb + 2*m*m*xb*xg - m*m*xg*xg + 2*m*xb*yb - 2*m*xg*yb - yb*yb) - m*yb + m*m*xb)/(m*m + 1);\ny = (yb - m*xb + m*xg + m*sqrt(R*R*m*m + R*R - m*m*xb*xb + 2*m*m*xb*xg - m*m*xg*xg + 2*m*xb*yb - 2*m*xg*yb - yb*yb))/(m*m + 1);"("xb"=w185, "yb"=w184, "xg"=w182, "R"=w179, "m"=0.0 ("input variable")) -> ("x"=w169:dbl, "y"=w168:dbl)
              n93 = Build Array(w169, w168) -> (w178:dbl[])
              n94 = Subtract(x=w167, y=w178) -> (x-y=w177:dbl[])
              n95 = Index Array(array=w177) -> (element #1=w176:dbl, element #2=w175:dbl)  [unwired: 2 in]
              n96 = Inverse Tangent (2 Input)(1:w176, 2:w175) -> (0:w170:dbl)
              n97 = property class="Robot"(reference=w173, "dest_orientation"=w170, "dest_x"=w169, "dest_y"=w168) -> (reference out=w186:refnum<class "Robot.lvclass">)  [unwired: 1 in, 1 out]
              n98 = call "DefendGoalTacticCheckStateChange.vi"("Game"=w191, "DefendGoalTactic in"=w194) -> ("States"=w195:T1)  [unwired: 7 in, 2 out]
            }
          }
        }
        frame "BlockPossibleShot" {
          n99 = disable-structure shown="Enabled" {
            disable-tunnel: w232 -> [w275 _]
            disable-tunnel: w231 -> [w261 w298]
            disable-tunnel: w229 -> [w251 w296]
            disable-tunnel: w230 -> [w239 w297]
            disable-tunnel: [_ w299] -> w228
            disable-tunnel: [_ w295] -> w227
            disable-tunnel: [_ w296] -> w225
            frame Disabled {
              n100 = property class="Game"(reference=w261) -> ("BallRef"=w249:refnum<class "Ball.lvclass">, "OffensiveTeam"=w276:refnum<class "Ally.lvclass">, "EnemyRef"=w277:refnum<class "Enemy.lvclass">, "FieldRef"=w250:refnum<class "Field.lvclass">, "Parameters.lvclass"=w279:refnum<class "Parameters.lvclass">)  [unwired: 1 in, 2 out]
              n101 = property class="Skillbook"(reference=w275) -> ("DefBallOrientSkill"=w238:refnum<class "DefBallOrientSkill.lvclass">, "DefBallEnemySkill"=w240:refnum<class "DefBallEnemySkill.lvclass">)  [unwired: 1 in, 2 out]
              n102 = property class="Field"(reference=w250) -> ("ourGoalPosition"=w259:dbl[], "goal_width"=w258:i32)  [unwired: 1 in, 2 out]
              n103 = property class="Ball"(reference=w249) -> (reference out=w236:refnum<class "Ball.lvclass">, "position(x,y)"=w265:dbl[])  [unwired: 1 in, 1 out]
              n104 = property class="Parameters.lvclass" props=["AttakingOurselves", "GoalieInFrontGoal"](reference=w279) -> ("AttakingOurselves"=w274:bool)  [unwired: 1 in, 3 out]
              n105 = Index Array(array=w259) -> (element=w245:dbl)  [unwired: 1 in]
              n106 = Subtract(x=w265, y=w259) -> (x-y=w273:dbl[])
              n107 = Divide(x=w258, y=2) -> (x/y=w256:dbl)
              n108 = Index Array(array=w273) -> (element #1=w254:dbl, element #2=w253:dbl)  [unwired: 2 in]
              n109 = Sign(1:w253) -> (0:w255:dbl)
              n110 = Inverse Tangent (2 Input)(1:w254, 2:w253) -> (0:w268:dbl)
              n111 = Absolute Value(x=w268) -> (abs(x)=w272:dbl)
              n112 = Select(t=w276, s=w274, f=w277) -> (s? t:f=w278:refnum<class "Team.lvclass">)
              n113 = Divide(x=3.141592653589793, y=4.0) -> (x/y=w269:dbl)
              n114 = Greater?(x=w272, y=w269) -> (0:w241:bool)
              n115 = property class="Team"(reference=w278) -> ("RobotRef"=w267:refnum<class "Robot.lvclass">[])  [unwired: 1 in, 2 out]
              n116 = call "findAllyOrEnemyRobotClosestToBall.vi"("Ally/Enemy Robots"=w267, "Ball"=w236) -> ("Robot"=w266:refnum<class "Robot.lvclass">)  [unwired: 5 in, 4 out]
              n117 = property class="Robot"(reference=w266) -> (reference out=w237:refnum<class "Robot.lvclass">, "position(x,y)"=w260:dbl[])  [unwired: 1 in, 1 out]
              n118 = call "IsAimingGoal.vi"("object in"=w251, "Game"=w261, "Robot position"=w260) -> ("Y aiming in goal coerced"=w246:dbl)  [unwired: 13 in, 3 out]
              n119 = Subtract(x=w265, y=w260) -> (x-y=w264:dbl[])
              n120 = Index Array(array=w264) -> (element #1=w262:dbl, element #2=w263:dbl)  [unwired: 2 in]
              n121 = Divide(x=w263, y=w262) -> (x/y=w252:dbl)
              n122 = call "robotOrientatedToBall.vi"("Robot"=w239, "BallRef"=w236) -> ("Orientation"=w234:dbl)  [unwired: 7 in, 2 out]
              n123 = call "coerceAngularCoef.vi"("object in"=w251, "Coef ang"=w252, "Field"=w250, "Ball"=w249) -> ("coerced(x)"=w244:dbl)  [unwired: 13 in, 2 out]
              n124 = formula code="x1 = (m*x_g - y_g + (y_g + m*sqrt(m*m*r*r + r*r - y_g*y_g))/(m*m + 1))/m;\nx2 = (m*x_g - y_g - (y_g + m*sqrt(m*m*r*r + r*r - y_g*y_g))/(m*m + 1))/m;"("m"=w244, "y_g"=w246, "x_g"=w245, "r"=w256, "s"=w255) -> ("x1"=w248:dbl, "x2"=w247:dbl)
              n125 = Max & Min(x=w248, y=w247) -> (max(x,y)=w243:dbl)  [unwired: 1 out]
              n126 = call "distanceRobotToBall.vi"("Robot"=w237, "Ball"=w236) -> ("Distance Robot To Ball"=w235:dbl)  [unwired: 7 in, 2 out]
              n127 = formula code="y = y_g+m*(x-x_g);"("m"=w244, "y_g"=w246, "x_g"=w245, "x"=w243) -> ("y"=w242:dbl)
              n128 = case shown="False" w241 {
                tunnel: w261 -> [w285 _]
                tunnel: w239 -> [w284 _]
                tunnel: w239 -> [_ w294]
                tunnel: [w287 w293] -> _
                tunnel: w243 -> [_ w292]
                tunnel: w242 -> [_ w291]
                tunnel: w235 -> [w282 _]
                tunnel: w240 -> [w289 _]
                tunnel: w238 -> [w283 _]
                tunnel: w234 -> [_ w290]
                frame False {
                  n129 = Less?(x=w282, y=400.0) -> (x < y?=w280:bool)
                  n130 = call "DefBallEnemySkill.vi"("Robot"=w284, "Game"=w285, "DefBallEnemySkill in"=w289) -> ("robot out"=w288:refnum<class "Robot.lvclass">)  [unwired: 6 in, 2 out]
                  n131 = call "DefBallOrientSkill.vi"("Robot"=w284, "Game"=w285, "DefBallOrientSkill in"=w283) -> ("Robot out"=w286:refnum<class "Robot.lvclass">)  [unwired: 6 in, 2 out]
                  n132 = Select(t=w286, s=w280, f=w288) -> (s? t:f=w287:refnum<class "Robot.lvclass">)
                }
                frame True {
                  n133 = property class="Robot"(reference=w294, "dest_x"=w292, "dest_y"=w291, "dest_orientation"=w290) -> (reference out=w293:refnum<class "Robot.lvclass">)  [unwired: 1 in, 1 out]
                }
              }
            }
            frame Enabled {
              n134 = call "BlockAngle.vi"("Game ref"=w298, "Robot in"=w297, "DefendGoalTactic in"=w296) -> ("Robot out"=w295:refnum<class "Robot.lvclass">)  [unwired: 6 in, 2 out]
              n135 = call "DefendGoalTacticCheckStateChange.vi"("Game"=w298, "DefendGoalTactic in"=w296) -> ("States"=w299:T1)  [unwired: 7 in, 2 out]
            }
          }
        }
        frame "Kick" {
          n136 = property class="Game"(reference=w319) -> ("NewParameters"=w328:T4)  [unwired: 1 in, 2 out]
          n137 = property class="Game"(reference=w319) -> ("FieldRef"=w316:refnum<class "Field.lvclass">, "BallRef"=w318:refnum<class "Ball.lvclass">)  [unwired: 1 in, 2 out]
          n138 = property class="Skillbook"(reference=w333) -> ("KickToSkill"=w334:refnum<class "KickToSkill.lvclass">)  [unwired: 1 in, 2 out]
          n139 = call "keeperTarget.vi"("Game in"=w319) -> ("pass"=w332:bool, "target"=w322:dbl[])  [unwired: 9 in]
          n140 = call "keeperStuck.vi"("Game"=w319, "Robot in"=w320, "DefendGoalTactic in"=w324) -> ("kepperStuck"=w305:bool)  [unwired: 6 in, 2 out]
          n141 = Unbundle By Name(w328) -> ("BadDribblerIDs"=w327:i32[])  [unwired: 1 out]
          n142 = property class="Field"(reference=w316) -> ("field_width"=w315:i32)  [unwired: 1 in, 2 out]
          n143 = property class="Ball"(reference=w318) -> ("x"=w317:dbl, "y"=w312:dbl)  [unwired: 1 in, 2 out]
          n144 = Divide(x=w315, y=2) -> (x/y=w313:dbl)
          n145 = Sign(1:w312) -> (0:w311:dbl)
          n146 = Multiply(x=w313, y=w311) -> (x*y=w310:dbl)
          n147 = Build Array(w317, w310) -> (w309:dbl[])
          n148 = Select(t=w309, s=w305, f=w322) -> (s? t:f=w321:dbl[])
          n149 = call "chooseKickTo.vi"("KickToSkill in"=w334, "Game in"=w319, "target gap"=dbl[] [0.0, 0.0], "Robot"=w320, "KickForce 0?"=FALSE, "use criteria?"=FALSE ("fixTarget"), "ForceInGame"=FALSE ("fixTarget"), "BadDribblerIDs"=w327, "pass?"=w332, "firstCall"=w329, "ChipKickInEnemyField"=TRUE, "Target"=w321) -> ("Robot out"=w307:refnum<class "Robot.lvclass">)  [unwired: 14 in, 1 out]
          n150 = call "DefendGoalTacticCheckStateChange.vi"("Game"=w319, "DefendGoalTactic in"=w324) -> ("States"=w308:T1)  [unwired: 7 in, 2 out]
          n151 = Select(t=20.0, s=w305, f=28.0) -> (s? t:f=w304:dbl)
          n152 = property class="Robot"(reference=w307, "kick_x"=w304, "kick_z"=1.0) -> (reference out=w306:refnum<class "Robot.lvclass">)  [unwired: 1 in, 1 out]
        }
        frame "GuardGoal" {
          n153 = property class="Game" props=["Parameters.lvclass", "BallRef", "FieldRef"](reference=w348) -> ("BallRef"=w342:refnum<class "Ball.lvclass">, "FieldRef"=w341:refnum<class "Field.lvclass">)  [unwired: 1 in, 3 out]
          n154 = property class="Field"(reference=w341) -> ("goal_width"=w338:i32, "ourGoalPosition"=w339:dbl[], "field_length"=w336:i32)  [unwired: 1 in, 2 out]
          n155 = disable-structure shown="Enabled" {
            disable-tunnel: [w366 w367] -> w347
            disable-tunnel: w346 -> [w365 _]
            disable-tunnel: [w364 w368] -> w345
            disable-tunnel: w342 -> [w363 _]
            disable-tunnel: [w362 w367] -> w340
            disable-tunnel: w339 -> [w355 _]
            disable-tunnel: w338 -> [w354 _]
            disable-tunnel: [0.0 ("kick_x") w367] -> w337
            disable-tunnel: w336 -> [_ w370]
            frame Disabled {
              # "Fica no Centroide do semicirculo"
              n156 = Index Array(array=w355) -> (element #1=w358:dbl, element #2=w362:dbl)  [unwired: 2 in]
              n157 = Divide(x=3, y=4) -> (x/y=w356:dbl)
              n158 = Multiply(x=w356, y=w354) -> (x*y=w361:dbl)
              n159 = Divide(x=w361, y=3.141592653589793) -> (x/y=w353:dbl)
              n160 = call "robotOrientatedToBall.vi"("Robot"=w365, "BallRef"=w363) -> ("Orientation"=w366:dbl)  [unwired: 7 in, 2 out]
              n161 = Add(x=w353, y=w358) -> (x+y=w364:dbl)
            }
            frame Enabled {
              w367 = 0.0
              n162 = Divide(x=w370, y=-2) -> (x/y=w368:dbl)
            }
          }
          n163 = call "DefendGoalTacticCheckStateChange.vi"("Game"=w348, "DefendGoalTactic in"=w349) -> ("States"=w350:T1)  [unwired: 7 in, 2 out]
          n164 = property class="Robot"(reference=w346, "dest_x"=w345, "dest_y"=w340, "dest_orientation"=w347, "kick_x"=w337, "kick_z"=w337) -> (reference out=w344:refnum<class "Robot.lvclass">)  [unwired: 1 in, 1 out]
        }
        frame "Exit" {
        }
      }
      n165 = feedback-in #2(w18) -> ()
      n166 = Or(x=w29, y=errorcluster {"status"=FALSE, "code"=0, "source"=""}) -> (x .or. y?=→"x .or. y?":bool)
      n167 = property class="DefendGoalTactic"(reference=w26, "States"=w18) -> (reference out=w25:refnum<class "DefendGoalTactic.lvclass">)  [unwired: 1 in, 1 out]
      n168 = property class="Robot"(reference=w20, "tactic"=tactics."DefendGoal", "keepDest"=w11) -> (reference out=w19:refnum<class "Robot.lvclass">)  [unwired: 1 in, 1 out]
    }
    frame Error {
    }
  }
  "error out" <- w7
  "Robot out" <- w5
  "DefendGoalTactic out" <- w2
